vi "File AI Stream Save.vi"(7 "DC Voltages Filename":path, 10 "Array":dbl[][](array[numeric]), 11 "Enable":bool) -> (2 "Time":string, 3 "new file path (Not A Path if cancelled)":path)   [LabVIEW 2012]
uses:
  <vilib>/Utility/file.llb/Write To Spreadsheet File (DBL).vi
  <vilib>/Utility/file.llb/Write To Spreadsheet File (string).vi
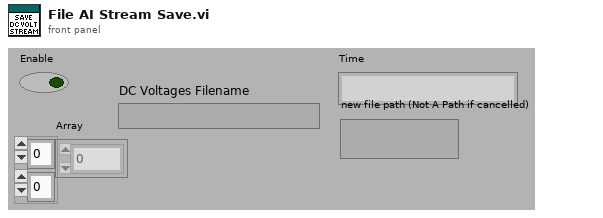
[diagram p1: front panel]
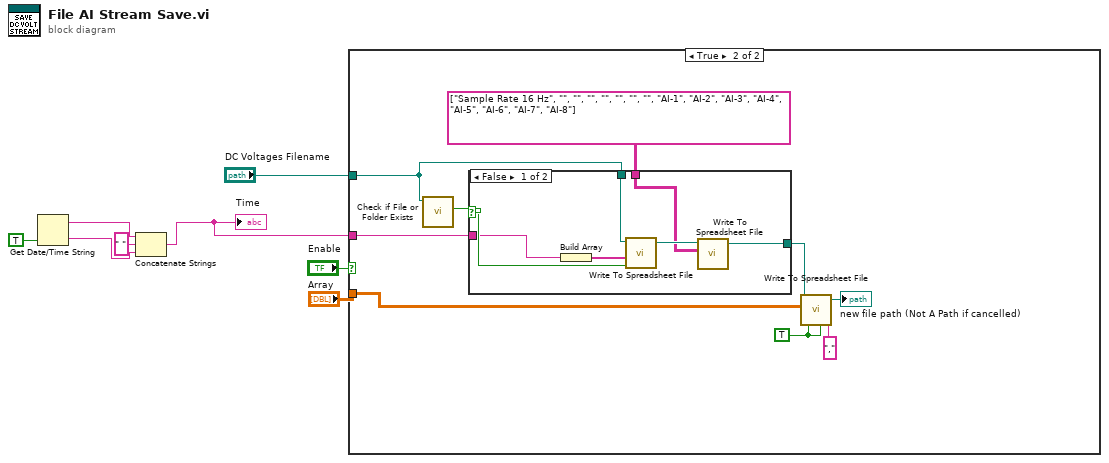
[diagram p0: block diagram]
diagram:
  n1 = Get Date/Time String(want seconds? (F)=TRUE) -> (date string=w3:string, time string=w2:string)  [unwired: 2 in]
  n2 = Concatenate Strings(w3, " " ("string"), w2) -> (w1:string)
  "Time" <- w1
  n3 = case shown="True" "Enable" {
    tunnel: "Array" -> [_ w17]
    tunnel: "DC Voltages Filename" -> [_ w13]
    tunnel: w1 -> [_ w12]
    frame False {
    }
    frame True {
      w15 = TRUE ("transpose? (no:F)")
      n4 = call <vilib>:"Check if File or Folder Exists.vi"("path"=w13) -> ("file or folder exists?"=w14:bool)  [unwired: 8 in, 2 out]
      n5 = case shown="False" w14 {
        selector: w14 -> [w24 _]
        tunnel: w13 -> [w22 w25]
        tunnel: w12 -> [w23 _]
        tunnel: string[][] [["Sample Rate 16 Hz", "", "", "", "", "", "", ""], ["AI-1", "AI-2", "AI-3", "AI-4", "AI-5", "AI-6", "AI-7", "AI-8"]] ("appended array") -> [w19 _]
        tunnel: [w20 w25] -> w10
        frame False {
          n6 = Build Array(w23) -> (w18:string[])
          n7 = call-poly <vilib>:"Write To Spreadsheet File.vi"("append to file? (new file:F)"=w24, "1D data"=w18, "file path (dialog if empty)"=w22) -> ("new file path (Not A Path if cancelled)"=w21:path)  [unwired: 5 in]
          n8 = call-poly <vilib>:"Write To Spreadsheet File.vi"("2D data"=w19, "file path (dialog if empty)"=w21) -> ("new file path (Not A Path if cancelled)"=w20:path)  [unwired: 6 in]
        }
        frame True {
        }
      }
      n9 = call-poly <vilib>:"Write To Spreadsheet File.vi"("delimiter (\\t)"="," ("delimiter (\\t)"), "transpose? (no:F)"=w15, "append to file? (new file:F)"=w15, "2D data"=w17, "file path (dialog if empty)"=w10) -> ("new file path (Not A Path if cancelled)"=→"new file path (Not A Path if cancelled)":path)  [unwired: 3 in]
    }
  }
